vi "WebService_Initialization.vi"(6 "LabVIEW Web Service":refnum<class "Web Service.lvclass">) -> ()   [LabVIEW 2024]
uses:
  <vilib>/wsapi/Web Service.lvclass
  DataTypes/AutoModeParameters.ctl
  DataTypes/ServoStatus.ctl
  DataTypes/OperationTypeForFunctionalGlobalVariable.ctl
  DataTypes/WebServiceStatus.ctl
panel:
  # "Use the web service input terminal to call the VIs on the Service subpalette of the Web Services palette. Do not remove it from the connector pane unless you don't need access to the palette."
  # "Any additional terminals added to the connector pane of a startup VI will be ignored."
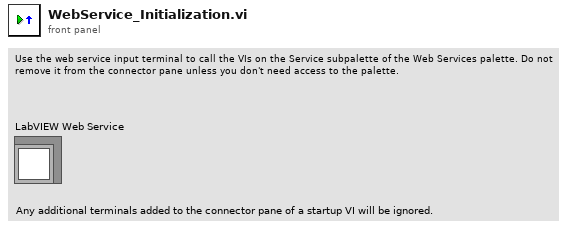
[diagram p1: front panel]
types:
  T1 = typedef "WebServiceStatus.ctl" = cluster{"isWebServiceShuttingDown":bool}
  T2 = typedef "OperationTypeForFunctionalGlobalVariable.ctl" = enum16{"GET", "SET"}
  T3 = typedef "ServoStatus.ctl" = cluster{"mode":string, "position":i16}
  T4 = typedef "AutoModeParameters.ctl" = cluster{"movementDirection":enum16{"TOWARDS_0_DEGREES", "TOWARDS_180_DEGREES"}, "frequency":dbl}
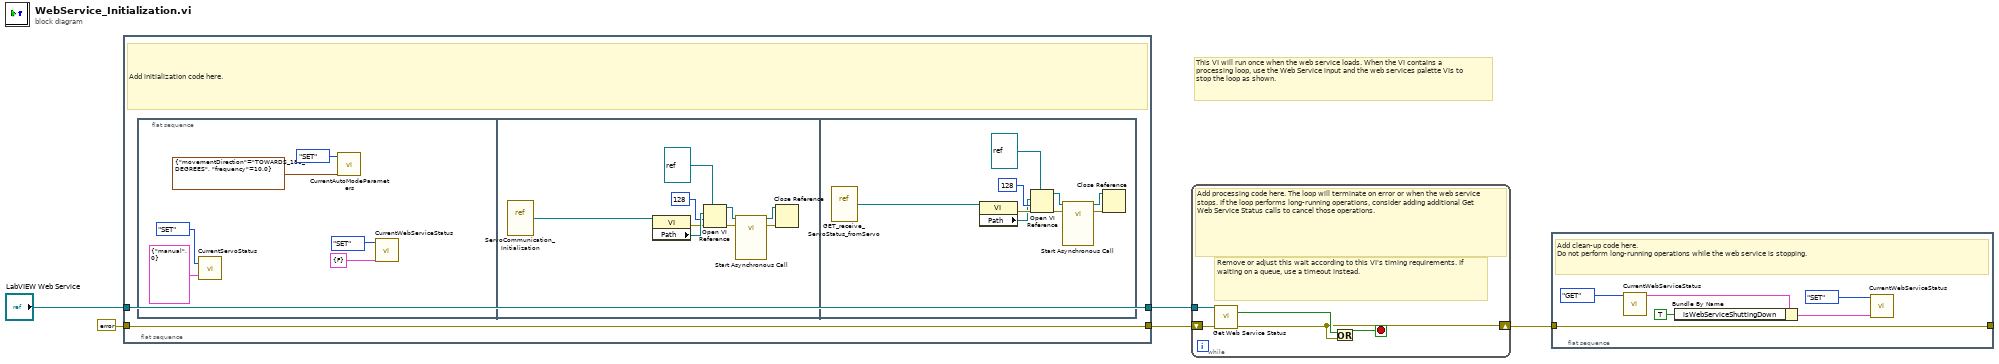
[diagram p0: block diagram]
diagram:
  # "This VI will run once when the web service loads. When the VI contains a processing loop, use the Web Service input and the web services palette VIs to stop the loop as shown."
  n1 = flat-sequence {
    tunnel: "LabVIEW Web Service" -> [w7]
    tunnel: [w7] -> w4
    tunnel: [w6] -> w3
    tunnel: errorcluster {"status"=FALSE, "code"=0, "source"=""} ("error constant") -> [w6]
    frame #0 {
      # "Add initialization code here."
      n2 = flat-sequence {
        frame #0 {
          n3 = call "CurrentServoStatus.vi"("New Servo Status"=T3 {"mode"="manual", "position"=0}, "Operation"=OperationTypeForFunctionalGlobalVariable."SET") -> ()  [unwired: 1 in, 1 out]
          n4 = call "CurrentAutoModeParameters.vi"("New Auto Mode Parameters"=T4 {"movementDirection"=enum."TOWARDS_180_DEGREES", "frequency"=10.0}, "Operation"=OperationTypeForFunctionalGlobalVariable."SET") -> ()  [unwired: 9 in, 1 out]
          n5 = call "CurrentWebServiceStatus.vi"("New WebService Status"=T1 {"isWebServiceShuttingDown"=FALSE}, "Operation"=OperationTypeForFunctionalGlobalVariable."SET") -> ()  [unwired: 9 in, 1 out]
        }
        frame #1 {
          n6 = vi-ref "ServoCommunication_Initialization.vi"() -> (w22:refnum<vi>)
          n7 = property class="VI"(reference=w22) -> (error out=w16:errorcluster, "Path"=w21:path)  [unwired: 1 in, 1 out]
          n8 = Open VI Reference(type specifier VI Refnum (for type only)=refnum<vi> refnum, vi path=w21, options=128, error in (no error)=w16) -> (vi reference=w14:refnum<vi>, error out=w17:errorcluster)  [unwired: 2 in]
          n9 = call-by-ref "Start Asynchronous Call"(reference=w14, error in=w17) -> (reference out=w19:refnum<vi>, error out=w18:errorcluster)  [unwired: 12 in]
          n10 = Close Reference(reference=w19, error in (no error)=w18) -> ()  [unwired: 1 out]
        }
        frame #2 {
          n11 = vi-ref "GET_receive_ServoStatus_fromServo.vi"() -> (w23:refnum<vi>)
          n12 = property class="VI"(reference=w23) -> (error out=w29:errorcluster, "Path"=w24:path)  [unwired: 1 in, 1 out]
          n13 = Open VI Reference(type specifier VI Refnum (for type only)=refnum<vi> refnum, vi path=w24, options=128, error in (no error)=w29) -> (vi reference=w31:refnum<vi>, error out=w28:errorcluster)  [unwired: 2 in]
          n14 = call-by-ref "Start Asynchronous Call"(reference=w31, error in=w28) -> (reference out=w26:refnum<vi>, error out=w27:errorcluster)  [unwired: 11 in]
          n15 = Close Reference(reference=w26, error in (no error)=w27) -> ()  [unwired: 1 out]
        }
      }
    }
  }
  n16 = while {
    tunnel: w4 -> [w35]
    shift-right: [w32] -> w1
    shift-left: w3 -> [w33]
    stop <- w34 stop-if-true
    # "Remove or adjust this wait according to this VI's timing requirements. If waiting on a queue, use a timeout instead."
    # "Add processing code here. The loop will terminate on error or when the web service stops. If the loop performs long-running operations, consider adding additional Get Web Service Status calls to cancel those operations."
    n17 = call <vilib>:"Get Web Service Status.vi"("LabVIEW Web Service"=w35, "error in (no error)"=w33) -> ("service stopping?"=w36:bool, "error out"=w32:errorcluster)  [unwired: 11 in, 1 out]
    n18 = Or(x=w36, y=w32) -> (x .or. y?=w34:bool)
  }
  n19 = flat-sequence {
    tunnel: [w42] -> _
    tunnel: w1 -> [w42]
    frame #0 {
      # "Add clean-up code here.\nDo not perform long-running operations while the web service is stopping."
      n20 = call "CurrentWebServiceStatus.vi"("Operation"=OperationTypeForFunctionalGlobalVariable."GET") -> ("Current WebService Status"=w40:T1)  [unwired: 10 in]
      n21 = Bundle By Name(cluster=w40, "isWebServiceShuttingDown"=TRUE) -> (w38:T1)
      n22 = call "CurrentWebServiceStatus.vi"("New WebService Status"=w38, "Operation"=OperationTypeForFunctionalGlobalVariable."SET") -> ()  [unwired: 9 in, 1 out]
    }
  }
